vi "Initial Recipe.vi"(8 "error in (no error)":errorcluster, 11 "Masterv2 in":refnum<class "Masterv2.lvclass">) -> (0 "error out":errorcluster, 3 "Masterv2 out":refnum<class "Masterv2.lvclass">)   [LabVIEW 2014, in "Main Libraryv2.lvlib" / "Masterv2.lvclass"]
uses:
  Master/Masterv2.lvclass
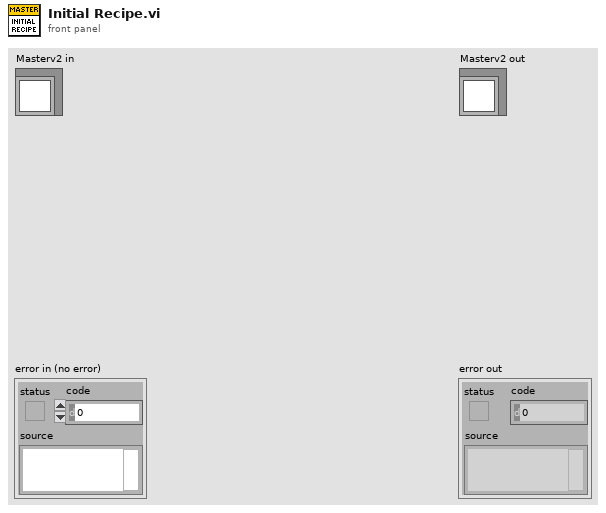
[diagram p1: front panel]
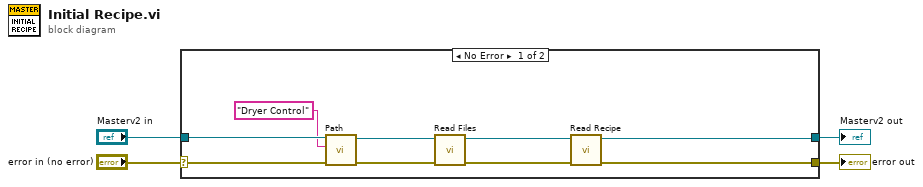
[diagram p0: block diagram]
diagram:
  n1 = case shown="No Error" "error in (no error)" {
    selector: "error in (no error)" -> [w13 w15]
    tunnel: [w10 w15] -> w3
    tunnel: [w6 w14] -> w1
    tunnel: "Masterv2 in" -> [w9 w14]
    frame No Error {
      n2 = call-dynamic "Path.vi"("error in (no error)"=w13, "pathname"="Dryer Control", "Masterv2 in"=w9) -> ("error out"=w12:errorcluster, "Masterv2 out"=w8:refnum<class "Masterv2.lvclass">)  [unwired: 7 in]
      n3 = call-dynamic "Read Files.vi"("error in (no error)"=w12, "Masterv2 in"=w8) -> ("error out"=w11:errorcluster, "Masterv2 out"=w7:refnum<class "Masterv2.lvclass">)  [unwired: 8 in]
      n4 = call-dynamic "Read Recipe.vi"("error in (no error)"=w11, "Masterv2 in"=w7) -> ("error out"=w10:errorcluster, "Masterv2 out"=w6:refnum<class "Masterv2.lvclass">)  [unwired: 8 in]
    }
    frame Error {
    }
  }
  "error out" <- w3
  "Masterv2 out" <- w1
